vi "Read.vi"(11 "AudioSummaryValue in":refnum<class "AudioSummaryValue.lvclass">) -> (2 "Audio Summary":T1)   [LabVIEW 2022 SP3, in "VMR Server.lvlib" / "AudioSummaryValue.lvclass"]
uses:
  AudioSummaryValue.lvclass
  AudioSummaryValue.lvclass/AudioSummaryValue.ctl
  VMR Server Shared/Channel.ctl
  VMR Server Shared/VMR Server Shared.lvlib
  VMR Server Shared/Audio Summary.ctl
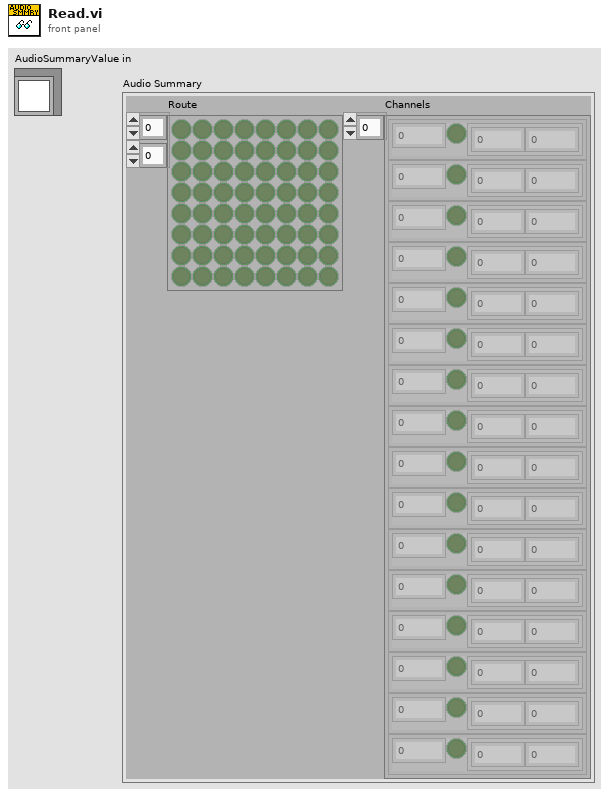
[diagram p1: front panel]
types:
  T1 = typedef "VMR Server Shared.lvlib/Audio Summary.ctl" = cluster{"Route":bool[][], "Channels":T2[]}
  T2 = typedef "VMR Server Shared.lvlib/Channel.ctl" = cluster{"Volume":dbl, "Muted":bool, "Levels":cluster{"L":dbl, "R":dbl}}
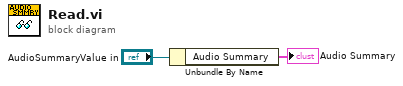
[diagram p0: block diagram]
diagram:
  n1 = Unbundle By Name("AudioSummaryValue in") -> ("Audio Summary"=→"Audio Summary":T1)
